vi "VCI_ReadBoardInfo.vi"(8 "error in (no error)":errorcluster caption="错误输入（无错误）", 10 "DevIndex":u32, 11 "DevType":T2=2 items=["USB-CAN"=2, "USB-CAN2"=3]) -> (0 "error out":errorcluster caption="错误输出", 2 "VCI_BOARD_INFO":T1, 3 "Return Val":T3=1 items=["OK"=1, "ERROR1"=0, "ERROR2"=-1])   [LabVIEW 2018, in "ControlCan.lvlib"]
uses:
  ControlCan.lvlib
  Return Val.ctl
  DevType.ctl
  VCI_BOARD_INFO.ctl
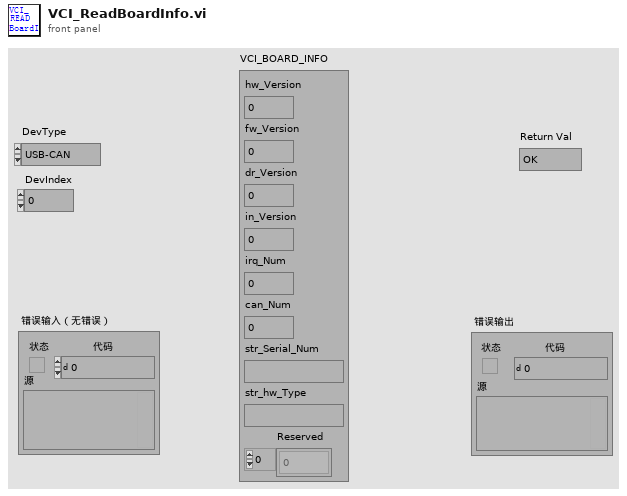
[diagram p1: front panel]
types:
  T1 = typedef "ControlCAN.lvlib/VCI_BOARD_INFO.ctl" = cluster{"hw_Version":u16, "fw_Version":u16, "dr_Version":u16, "in_Version":u16, "irq_Num":u16, "can_Num":u8, "str_Serial_Num":string, "str_hw_Type":string, "Reserved":u8[]}
  T2 = typedef "ControlCAN.lvlib/DevType.ctl" = u32
  T3 = typedef "ControlCAN.lvlib/Return Val.ctl" = i32
  T4 = typedef "ControlCAN.lvlib/VCI_BOARD_INFO_1.ctl" = cluster{"hw_Version":u16, "fw_Version":u16, "dr_Version":u16, "in_Version":u16, "irq_Num":u16, "can_Num":u8, "str_Serial_Num 0":u8, "str_Serial_Num 1":u8, "str_Serial_Num 2":u8, "str_Serial_Num 3":u8, "str_Serial_Num 4":u8, "str_Serial_Num 5":u8, "str_Serial_Num 6":u8, "str_Serial_Num 7":u8, "str_Serial_Num 8":u8, "str_Serial_Num 9":u8, "str_Serial_Num 10":u8, "str_Serial_Num 11":u8, "str_Serial_Num 12":u8, "str_Serial_Num 13":u8, "str_Serial_Num 14":u8, "str_Serial_Num 15":u8, "str_Serial_Num 16":u8, "str_Serial_Num 17":u8, "str_Serial_Num 18":u8, "str_Serial_Num 19":u8, "str_hw_Type 0":u8, "str_hw_Type 1":u8, "str_hw_Type 2":u8, "str_hw_Type 3":u8, "str_hw_Type 4":u8, "str_hw_Type 5":u8, "str_hw_Type 6":u8, "str_hw_Type 7":u8, "str_hw_Type 8":u8, "str_hw_Type 9":u8, "str_hw_Type 10":u8, "str_hw_Type 11":u8, "str_hw_Type 12":u8, "str_hw_Type 13":u8, "str_hw_Type 14":u8, "str_hw_Type 15":u8, "str_hw_Type 16":u8, "str_hw_Type 17":u8, "str_hw_Type 18":u8, "str_hw_Type 19":u8, "str_hw_Type 20":u8, "str_hw_Type 21":u8, "str_hw_Type 22":u8, "str_hw_Type 24":u8, "str_hw_Type 25":u8, "str_hw_Type 26":u8, "str_hw_Type 27":u8, "str_hw_Type 28":u8, "str_hw_Type 29":u8, "str_hw_Type 30":u8, "str_hw_Type 31":u8, "str_hw_Type 32":u8, "str_hw_Type 33":u8, "str_hw_Type 34":u8, "str_hw_Type 35":u8, "str_hw_Type 36":u8, "str_hw_Type 37":u8, "str_hw_Type 38":u8, "str_hw_Type 39":u8, "Reserved 0":u8, "Reserved 1":u8, "Reserved 2":u8, "Reserved 3":u8}
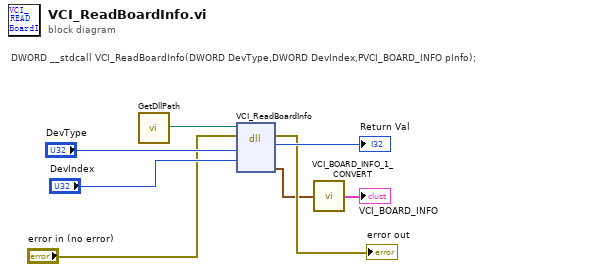
[diagram p0: block diagram]
diagram:
  # "DWORD __stdcall VCI_ReadBoardInfo(DWORD DevType,DWORD DevIndex,PVCI_BOARD_INFO pInfo);"
  n1 = call "GetDllPath.vi"() -> ("DllPath"=w1:path)  [unwired: 1 in]
  n2 = dll-call lib="?" fn="VCI_ReadBoardInfo"(path in=w1, error in="error in (no error)", "DevType"="DevType", "DevIndex"="DevIndex") -> (error out=→"error out":errorcluster, "ReturnVal"=→"Return Val":i32, "VCI_BOARD_INFO_1"=w3:T4)  [unwired: 4 in, 1 out]
  n3 = call "VCI_BOARD_INFO_1_CONVERT.vi"("VCI_BOARD_INFO_1"=w3) -> ("VCI_BOARD_INFO"=→"VCI_BOARD_INFO":T1)
